vi "最小公倍数.vi"(1 "采样率":i32[](array[numeric])) -> (0 "最小公倍数 2":i32)   [LabVIEW 2014]
panel:
  in  "b":i32
  in  "a":i32
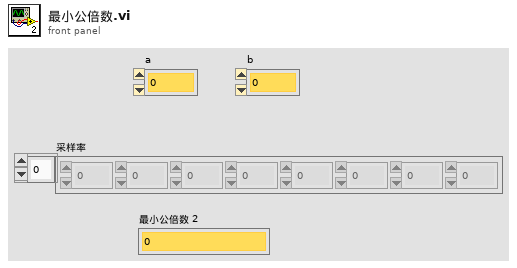
[diagram p1: front panel]
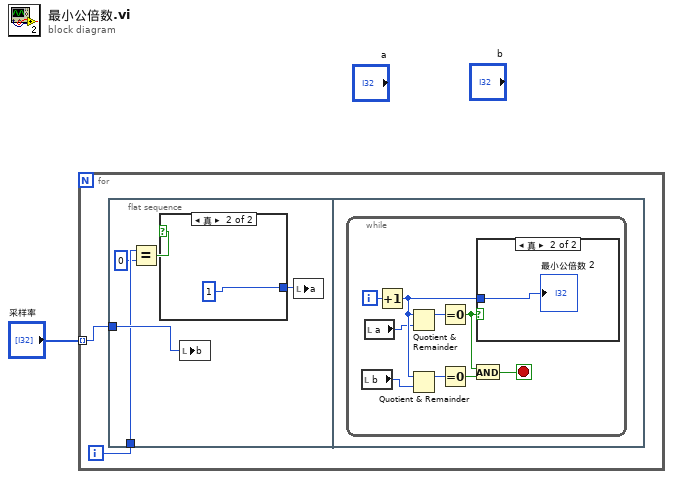
[diagram p0: block diagram]
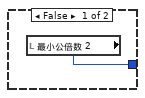
[diagram p2: hidden frame]
diagram:
  n1 = for {
    tunnel: "采样率" -> [w3] mode=indexing
    i -> [w2]
    n2 = flat-sequence {
      tunnel: w3 -> [w8]
      tunnel: w2 -> [w6]
      frame #0 {
        n3 = Equal?(x=w6, y=0) -> (x = y?=w7:bool)
        n4 = case shown="真" w7 {
          tunnel: [w9 i16 1 ("a")] -> w4
          frame False {
            n5 = local read "最小公倍数 2"() -> (w9:i32)
          }
          frame True {
          }
        }
        n6 = local write "b"(w8) -> ()
        n7 = local write "a"(w4) -> ()
      }
      frame #1 {
        n8 = while {
          i -> [w18]
          stop <- w13 stop-if-true
          n9 = local read "b"() -> (w12:i32)
          n10 = local read "a"() -> (w11:i32)
          n11 = Increment(x=w18) -> (x+1=w17:i32)
          n12 = Quotient & Remainder(x=w17, y=w11) -> (x-y*floor(x/y)=w16:i32)  [unwired: 1 out]
          n13 = Quotient & Remainder(x=w17, y=w12) -> (x-y*floor(x/y)=w15:i32)  [unwired: 1 out]
          n14 = Equal To 0?(x=w16) -> (x = 0?=w14:bool)
          n15 = Equal To 0?(x=w15) -> (x = 0?=w19:bool)
          n16 = And(x=w14, y=w19) -> (x .and. y?=w13:bool)
          n17 = case shown="真" w14 {
            tunnel: w17 -> [_ w20]
            frame False {
            }
            frame True {
              "最小公倍数 2" <- w20
            }
          }
        }
      }
    }
  }
